vi "Filter TX signals.vi"(9 "Pulse Shaping Filter Coefficients":dbl[](array[numeric]) format="%.2f", 10 "Samples Per Symbol (16)":i32=16, 11 "Symbols":cdb[](array[numeric]) format="%.2f") -> (3 "Filtered Samples":cdb[](array[numeric]) format="%.2f")   [LabVIEW 2011]
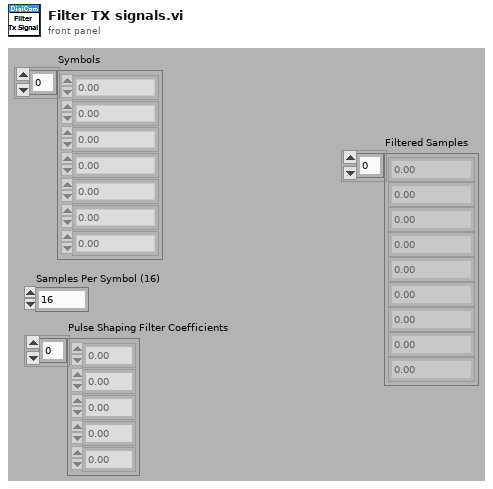
[diagram p1: front panel]
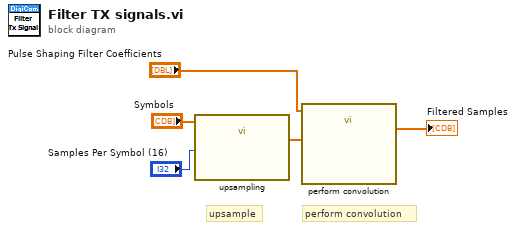
[diagram p0: block diagram]
diagram:
  # "perform convolution"
  # "upsample"
  n1 = call "upsampling.vi"("L"="Samples Per Symbol (16)", "x"="Symbols") -> ("y"=w3:cdb[])
  n2 = call "perform convolution.vi"("Sample stream"=w3, "Pulse Shaping Filter Coefficients"="Pulse Shaping Filter Coefficients") -> ("Filtered sample stream"=→"Filtered Samples":cdb[])  [unwired: 9 in]
